vi "Configure Level (Electrical Attenuation).vi"(0 "VISA resource name":refnum<visa-resource-name>, 1 "Auto Mechanical Attenuation (T: Enable)":bool=TRUE, 2 "Mechanical Attenuation Step (0: 2 dB)":i32(ring) items=["2", "10"], 3 "Manual Mechanical Attenuation (10 dB)":dbl=10.0, 5 "Reference Level (0 dBm)":dbl, 7 "Reference Level Offset (0 dB)":dbl, 9 "Amplitude Units (0: dBm)":i32(ring) items=["dBm", "dBmV", "dBmA", "W", "V", "A", "dBuV", "dBuA"], 11 "error in (no error)":errorcluster, 12 "Enable Electrical Attenuation (F: Disable)":bool, 13 "Electrical Attenuation (0 dB)":dbl) -> (4 "VISA resource name out":refnum<visa-resource-name>, 15 "error out":errorcluster)   [LabVIEW 2018, in "Agilent MXA Series.lvlib"]
doc: "Configures the vertical settings of the spectrum analyzer with Electrical Attenuation."
uses:
  Agilent MXA Series.lvlib
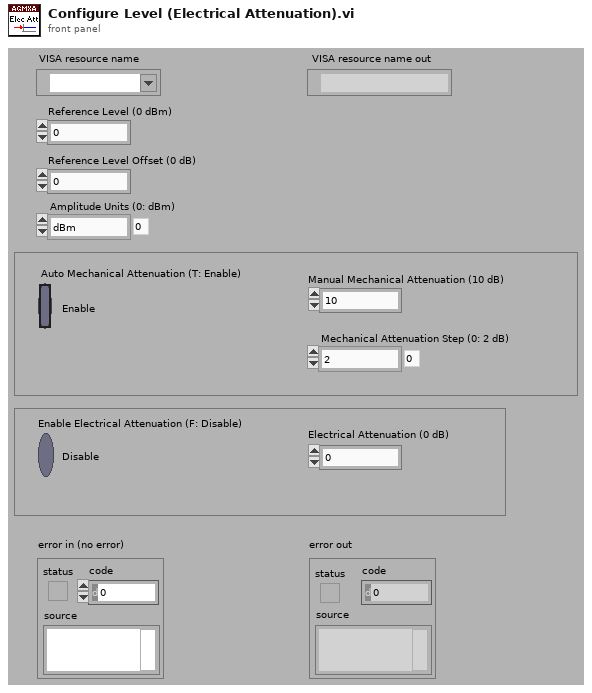
[diagram p1: front panel]
types:
  T1 = typedef "Agilent MXA Series.lvlib/Extended User Data.ctl" = cluster{"Measurement Type":i32, "Agilent MXA/EXA Model":i32}
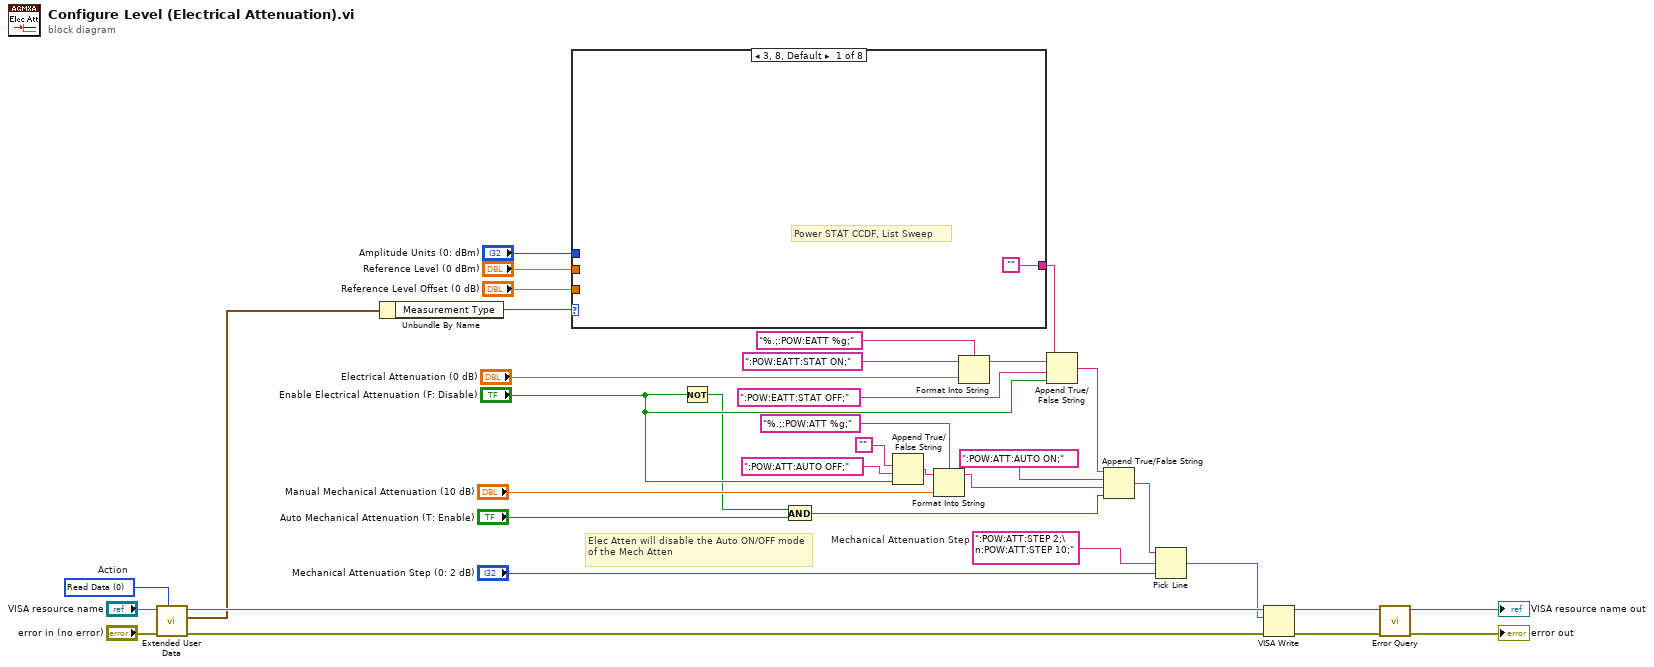
[diagram p0: block diagram]
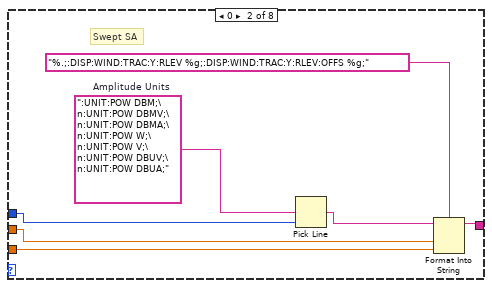
[diagram p2: hidden frame]
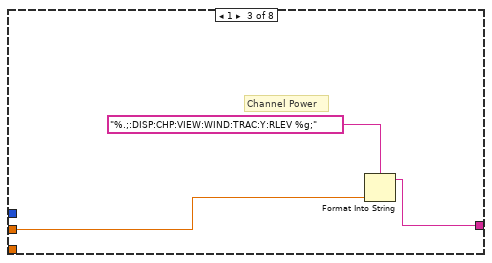
[diagram p3: hidden frame]
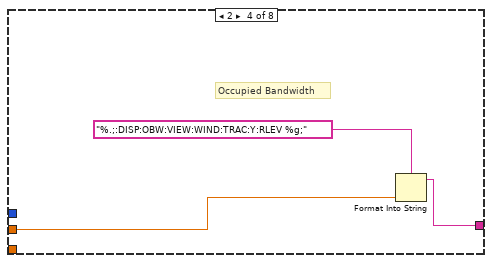
[diagram p4: hidden frame]
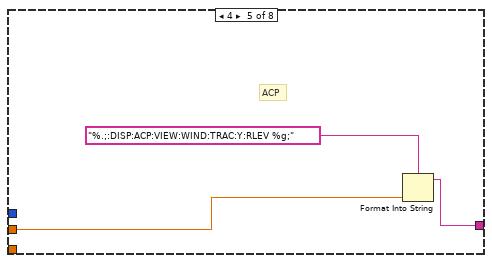
[diagram p5: hidden frame]
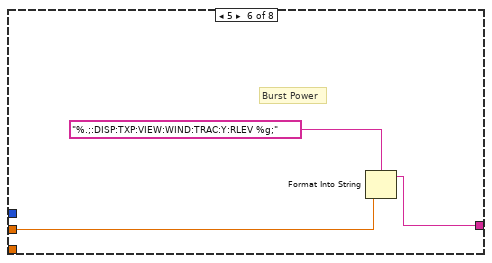
[diagram p6: hidden frame]
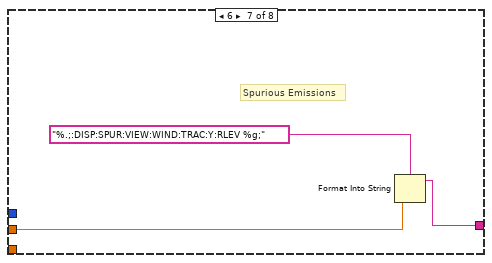
[diagram p7: hidden frame]
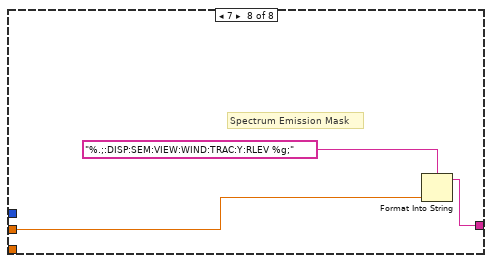
[diagram p8: hidden frame]
diagram:
  w14 = 0 items=["Read Data", "Write Data", "Clear Data", "Clear ALL Data"]  # Action
  w25 = ":POW:ATT:STEP 2;\n:POW:ATT:STEP 10;"  # Mechanical Attenuation Step
  # "Elec Atten will disable the Auto ON/OFF mode of the Mech Atten"
  n1 = call "Extended User Data.vi"("Action (1:Write Data)"=w14, "Error In (no error)"="error in (no error)", "VISA resource name in"="VISA resource name") -> ("Error Out"=w29:errorcluster, "User Data Out"=w19:T1, "VISA resource name out"=w30:refnum<visa-resource-name>)  [unwired: 6 in]
  n2 = Unbundle By Name(w19) -> ("Measurement Type"=w18:i32)
  n3 = case shown="3, 8, Default" w18 {
    tunnel: "Reference Level (0 dBm)" -> [_ w40 w46 w49 w52 w55 w58 w61]
    tunnel: "Reference Level Offset (0 dB)" -> [_ w39 _ _ _ _ _ _]
    tunnel: "Amplitude Units (0: dBm)" -> [_ w41 _ _ _ _ _ _]
    tunnel: ["" w38 w45 w48 w51 w54 w57 w60] -> w3
    frame 3, 8, Default {
      # "Power STAT CCDF, List Sweep"
    }
    frame 0 {
      w43 = ":UNIT:POW DBM;\n:UNIT:POW DBMV;\n:UNIT:POW DBMA;\n:UNIT:POW W;\n:UNIT:POW V;\n:UNIT:POW DBUV;\n:UNIT:POW DBUA;"  # Amplitude Units
      # "Swept SA"
      n4 = Pick Line(multi-line string=w43, line index=w41) -> (output string=w42:string)  [unwired: 1 in]
      n5 = Format Into String(format string="%.;:DISP:WIND:TRAC:Y:RLEV %g;:DISP:WIND:TRAC:Y:RLEV:OFFS %g;", initial string=w42, w40, w39) -> (resulting string=w38:string)  [unwired: 1 in, 1 out]
    }
    frame 1 {
      # "Channel Power"
      n6 = Format Into String(format string="%.;:DISP:CHP:VIEW:WIND:TRAC:Y:RLEV %g;", w46) -> (resulting string=w45:string)  [unwired: 2 in, 1 out]
    }
    frame 2 {
      # "Occupied Bandwidth"
      n7 = Format Into String(format string="%.;:DISP:OBW:VIEW:WIND:TRAC:Y:RLEV %g;", w49) -> (resulting string=w48:string)  [unwired: 2 in, 1 out]
    }
    frame 4 {
      # "ACP"
      n8 = Format Into String(format string="%.;:DISP:ACP:VIEW:WIND:TRAC:Y:RLEV %g;", w52) -> (resulting string=w51:string)  [unwired: 2 in, 1 out]
    }
    frame 5 {
      # "Burst Power"
      n9 = Format Into String(format string="%.;:DISP:TXP:VIEW:WIND:TRAC:Y:RLEV %g;", w55) -> (resulting string=w54:string)  [unwired: 2 in, 1 out]
    }
    frame 6 {
      # "Spurious Emissions"
      n10 = Format Into String(format string="%.;:DISP:SPUR:VIEW:WIND:TRAC:Y:RLEV %g;", w58) -> (resulting string=w57:string)  [unwired: 2 in, 1 out]
    }
    frame 7 {
      # "Spectrum Emission Mask"
      n11 = Format Into String(format string="%.;:DISP:SEM:VIEW:WIND:TRAC:Y:RLEV %g;", w61) -> (resulting string=w60:string)  [unwired: 2 in, 1 out]
    }
  }
  n12 = Not(x="Enable Electrical Attenuation (F: Disable)") -> (.not. x?=w5:bool)
  n13 = And(x=w5, y="Auto Mechanical Attenuation (T: Enable)") -> (x .and. y?=w13:bool)
  n14 = Append True/False String(1:"Enable Electrical Attenuation (F: Disable)", 2:":POW:ATT:AUTO OFF;" ("initial string"), 3:"") -> (0:w9:string)  [unwired: 1 in]
  n15 = Format Into String(format string="%.;:POW:ATT %g;", initial string=w9, "Manual Mechanical Attenuation (10 dB)") -> (resulting string=w11:string)  [unwired: 1 in, 1 out]
  n16 = Format Into String(format string="%.;:POW:EATT %g;", initial string=":POW:EATT:STAT ON;", "Electrical Attenuation (0 dB)") -> (resulting string=w1:string)  [unwired: 1 in, 1 out]
  n17 = Append True/False String(1:"Enable Electrical Attenuation (F: Disable)", 2:":POW:EATT:STAT OFF;" ("true string"), 3:w1, 4:w3) -> (0:w6:string)
  n18 = Append True/False String(1:w13, 2:w11, 3:":POW:ATT:AUTO ON;" ("true string"), 4:w6) -> (0:w12:string)
  n19 = Pick Line(string ("")=w12, multi-line string=w25, line index="Mechanical Attenuation Step (0: 2 dB)") -> (output string=w2:string)
  n20 = VISA Write(VISA resource name=w30, write buffer=w2, error in (no error)=w29) -> (VISA resource name out=w36:refnum<visa-resource-name>, error out=w34:errorcluster)  [unwired: 1 out]
  n21 = call "Error Query.vi"("error in (no error)"=w34, "VISA resource name"=w36) -> ("error out"=→"error out":errorcluster, "VISA resource name out"=→"VISA resource name out":refnum<visa-resource-name>)  [unwired: 6 in, 2 out]
